vi "Turn Crank.vi"(0 "reference in":refnum<class "State.lvclass">, 5 "error in (no error)":errorcluster) -> (14 "reference out":refnum<class "State.lvclass">, 19 "error out":errorcluster)   [LabVIEW 2013, in "State.lvclass"]
uses:
  State.lvclass
  <vilib>/addons/_AddQ/G#Object/G#Object.lvclass
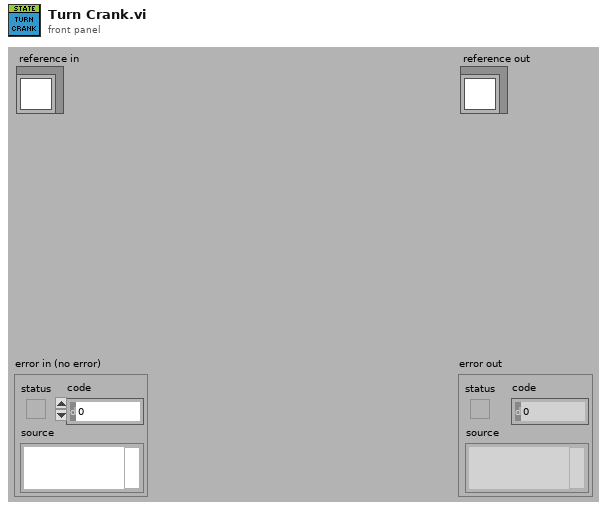
[diagram p1: front panel]
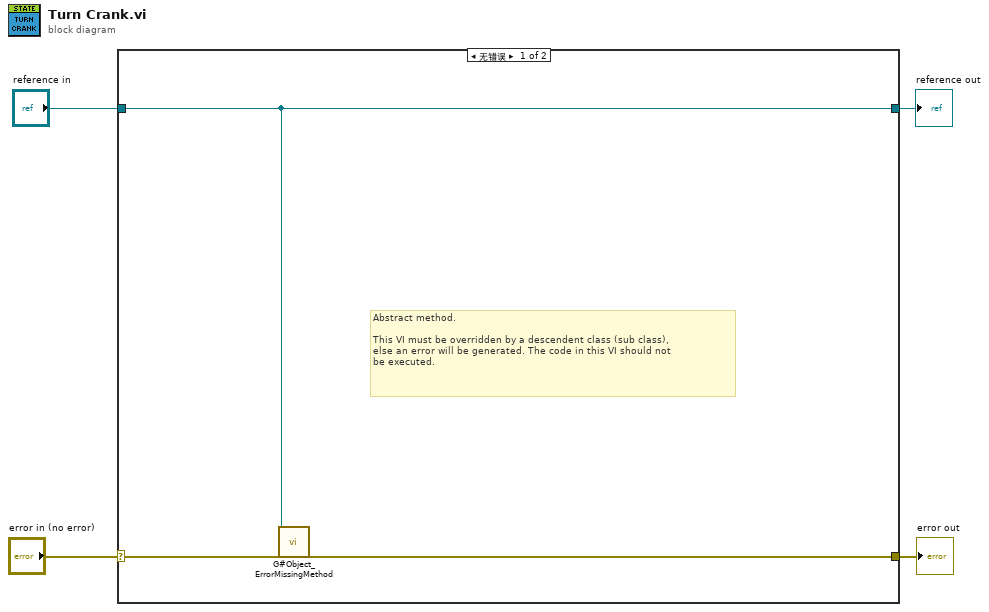
[diagram p0: block diagram]
diagram:
  n1 = case shown="无错误" "error in (no error)" {
    selector: "error in (no error)" -> [w7 w9]
    tunnel: [w6 w9] -> w3
    tunnel: [w5 w8] -> w1
    tunnel: "reference in" -> [w5 w8]
    frame No Error {
      # "Abstract method.\n\nThis VI must be overridden by a descendent class (sub class),\nelse an error will be generated. The code in this VI should not\nbe executed."
      n2 = call <vilib>:"G#Object_ErrorMissingMethod.vi"("reference in"=w5, "error in (no error)"=w7) -> ("error out"=w6:errorcluster)  [unwired: 16 in, 1 out]
    }
    frame Error {
    }
  }
  "error out" <- w3
  "reference out" <- w1
